vi "Apply New Configuration File.vi"(8 "error in (no error)":errorcluster, 9 "MD5 Hash In":string, 10 "File Path In":path, 11 "CD Ref In":T1=18446744073709551615 format="%.0x") -> (0 "error out":errorcluster, 1 "MD5 Hash Out":string, 2 "File Path Out":path, 3 "Last File content":string)   [LabVIEW 2021, in "Modbus System Explorer.lvlib"]
uses:
  Modbus System Explorer.lvlib
  <vilib>/NI VeriStand/Custom Device API/Custom Device Item Ref.ctl
  Shared/3_But_Dlg_Symbol.ctl
  Shared/Modbus GUID Lookup.vi
  <vilib>/NI VeriStand/Custom Device Tools/Custom Device Utility Library/NI VeriStand - Search for All Items by GUID.vi
  Glyphs/Modbus Dialog Messages.vi
  Glyphs/Modbus Property Names.vi
  <vilib>/NI VeriStand/Custom Device API/Get Item Property (String).vi
  <vilib>/NI VeriStand/Custom Device API/Get Item Property (Path).vi
  <vilib>/NI VeriStand/Custom Device API/Set Item Property (Variant).vi
  <vilib>/NI VeriStand/Custom Device API/Set Item Property (Path).vi
  <vilib>/NI VeriStand/Custom Device API/Set Item Property (String).vi
  Shared/Modbus Shared.lvlib
  <vilib>/NI VeriStand/Custom Device API/Custom Device API.lvlib
  XML Deserializer/XML VIs/API/XML_Deserializer.lvlib
  <vilib>/NI VeriStand/Custom Device Tools/Custom Device Utility Library/Custom Device Utility Library.lvlib
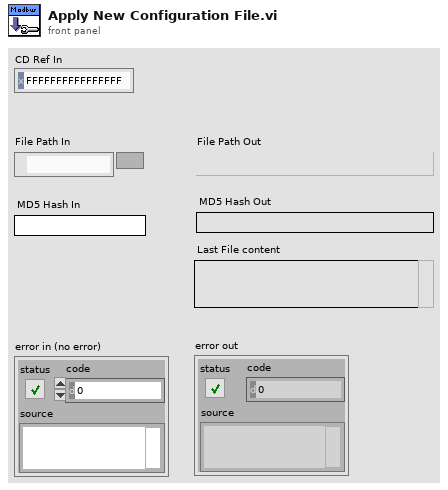
[diagram p1: front panel]
types:
  T1 = typedef "Custom Device API.lvlib/Custom Device Item Ref.ctl" = u64
  T2 = typedef "Modbus Shared.lvlib/3_But_Dlg_Symbol.ctl" = enum16{"Information", "Help", "Warning", "Error"}
  T3 = typedef "Modbus Shared.lvlib/Modbus_General_Settings.ctl" = cluster{"Communication_Type":T4, "Modbus_Type":T5, "Read_Write_Loop_Period":i64, "TCP Settings":cluster{"TCP_Settings_Port":u16, "TCP_Settings_IP_Timeout":u32, "TCP_Settings_IP_Slave_Address":string}, "Serial Settings":cluster{"Serial_Settings_Flow_Control":T6, "Serial_Settings_Baud_Rate":u32, "Serial_Settings_Parity":T7, "Serial_Settings_Resource_Name":string, "Serial_Settings_Serial_Type":T8, "Serial_Settings_Unit_ID":u8}}
  T4 = typedef "Modbus Shared.lvlib/Modbus_Communication_Type.ctl" = i32
  T5 = typedef "Modbus Shared.lvlib/Modbus_Type.ctl" = i32
  T6 = typedef "Modbus Shared.lvlib/Modbus_Serial_Settings_Flow_Control.ctl" = i32
  T7 = typedef "Modbus Shared.lvlib/Modbus_Serial_Settings_Parity.ctl" = i32
  T8 = typedef "Modbus Shared.lvlib/Modbus_Serial_Settings_Serial_Type.ctl" = i32
  T9 = typedef "Modbus Shared.lvlib/Modbus_Items.ctl" = cluster{"Modbus Type":T10, "Base Name":string, "Starting Address":u16, "Quantity":u16}
  T10 = typedef "Modbus Shared.lvlib/Modbus_Item_Type.ctl" = enum16{"Read Coils", "Read Discrete Inputs", "Read Holding Registers", "Read Input Registers", "Write Multiple Coils", "Write Multiple Holding Registers", "Write Single Coil", "Write Single Holding Register", "Write Multiple Discrete Inputs", "Write Multiple Input Registers"}
  T11 = typedef "Modbus Shared.lvlib/Channels Ref.ctl" = cluster{"Array of Refs":T1[]}
  T12 = typedef "Modbus Shared.lvlib/FIFO Indexes.ctl" = cluster{"FIFO Indexes":i32[], "FIFO Buffer":T13}
  T13 = typedef "Custom Device API.lvlib/Custom Device Channel Type.ctl" = enum16{"Input", "Output"}
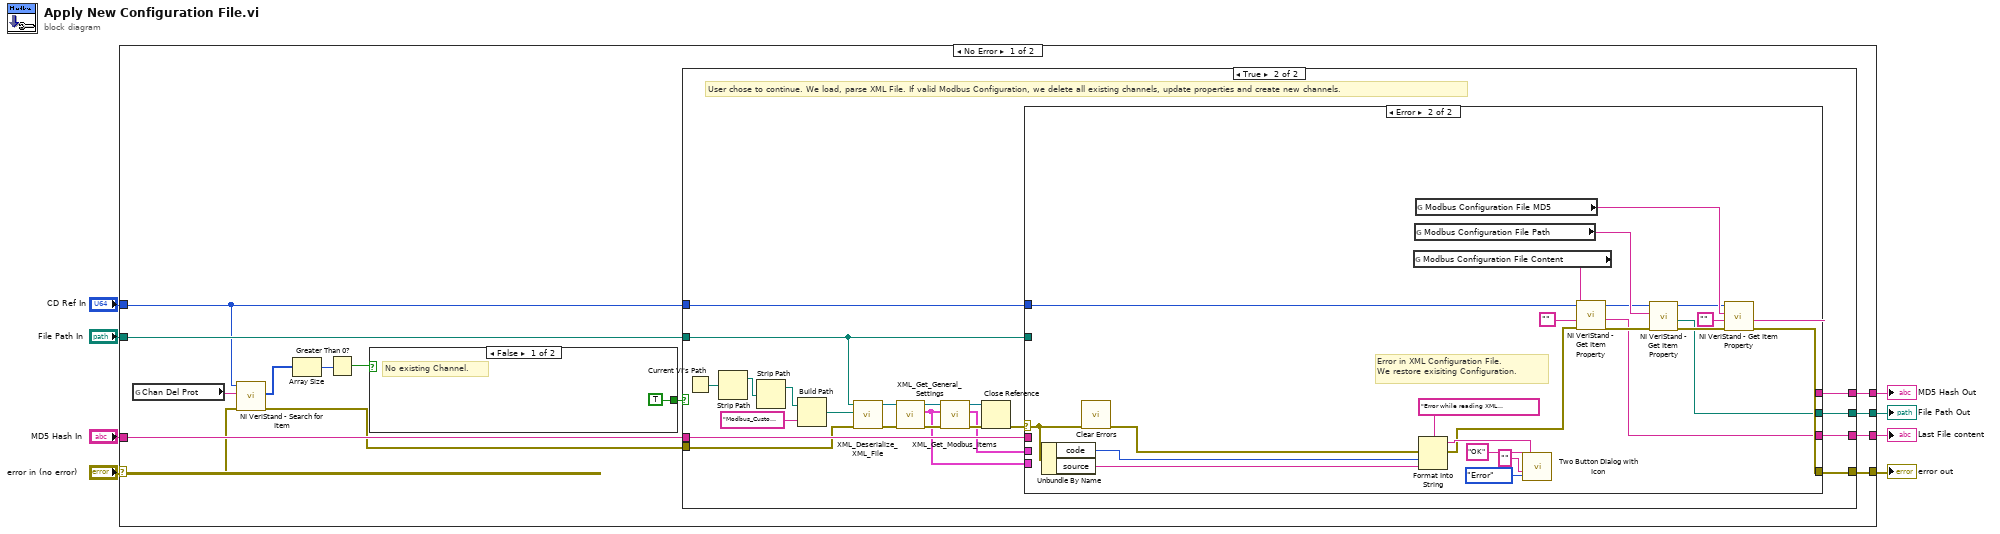
[diagram p0: block diagram]
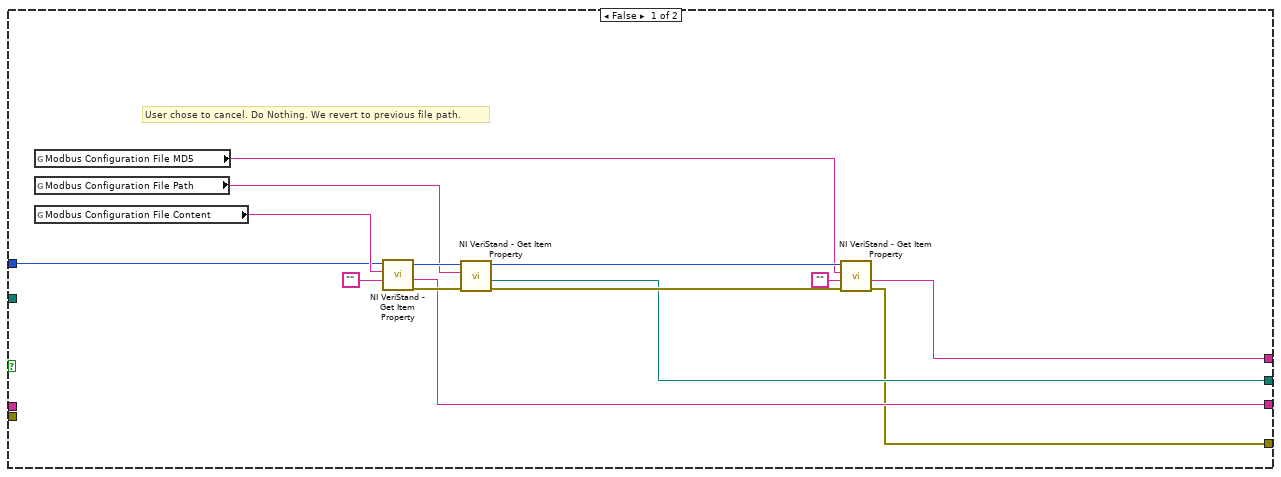
[diagram p2: hidden frame]
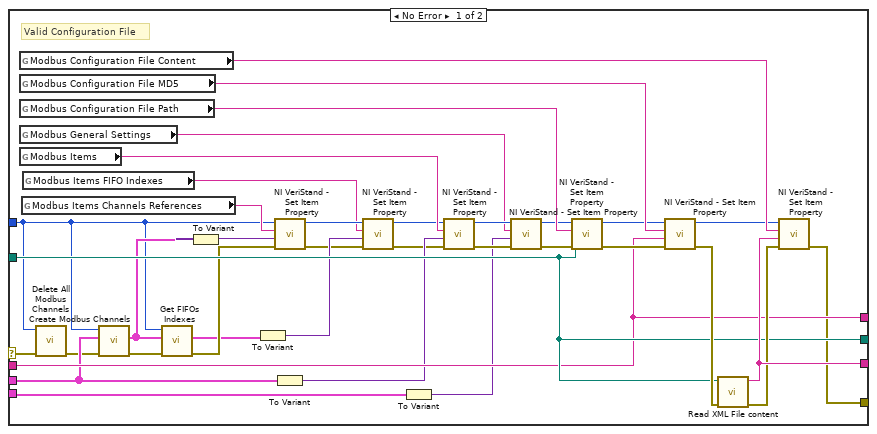
[diagram p3: hidden frame]
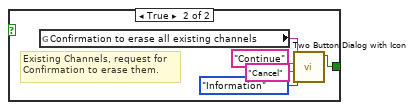
[diagram p4: hidden frame]
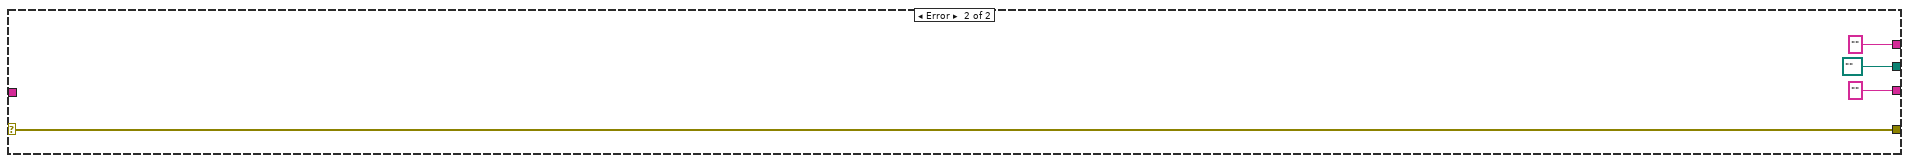
[diagram p5: hidden frame]
diagram:
  n1 = case shown="No Error" "error in (no error)" {
    selector: "error in (no error)" -> [w13 w129]
    tunnel: [w17 w129] -> w7
    tunnel: "CD Ref In" -> [w14 _]
    tunnel: "File Path In" -> [w21 _]
    tunnel: [w20 "" ("MD5 Hash In")] -> w4
    tunnel: [w19 path "" ("File Path In")] -> w3
    tunnel: [w18 "" ("XML File content")] -> w2
    tunnel: "MD5 Hash In" -> [w16 _]
    frame No Error {
      n2 = global read "Modbus GUID Lookup.vi" "Chan Del Prot"() -> (w15:string)
      n3 = call-poly <vilib>:"NI VeriStand - Search for Item.vi"("error in"=w13, "Item GUID"=w15, "Section Ref in"=w14) -> ("error out"=w9:errorcluster, "Item Refs"=w12:T1[])  [unwired: 5 in, 2 out]
      n4 = Array Size(array=w12) -> (size(s)=w11:i32)
      n5 = Greater Than 0?(x=w11) -> (x > 0?=w10:bool)
      n6 = case shown="False" w10 {
        tunnel: [TRUE ("T button?") w124] -> w22
        frame False {
          # "No existing Channel."
        }
        frame True {
          # "Existing Channels, request for\nConfirmation to erase them."
          n7 = global read "Modbus Dialog Messages.vi" "Confirmation to erase all existing channels"() -> (w123:string)
          n8 = call "Two Button Dialog with Icon.vi"("Symbol"=3_But_Dlg_Symbol."Information", "F button name (\"Cancel\")"="Cancel" ("F button name (\"Cancel\")"), "T button name (\"OK\")"="Continue" ("T button name (\"OK\")"), "Message"=w123) -> ("T Button?"=w124:bool)  [unwired: 7 in]
        }
      }
      n9 = case shown="True" w22 {
        tunnel: w14 -> [w28 w55]
        tunnel: w21 -> [_ w45]
        tunnel: [w27 w53] -> w20
        tunnel: [w26 w54] -> w19
        tunnel: [w25 w58] -> w18
        tunnel: [w24 w56] -> w17
        tunnel: w16 -> [_ w57]
        tunnel: w9 -> [_ w37]
        frame False {
          # "User chose to cancel. Do Nothing. We revert to previous file path."
          n10 = global read "Modbus Property Names.vi" "Modbus Configuration File MD5"() -> (w31:string)
          n11 = global read "Modbus Property Names.vi" "Modbus Configuration File Path"() -> (w32:string)
          n12 = global read "Modbus Property Names.vi" "Modbus Configuration File Content"() -> (w30:string)
          n13 = call-poly <vilib>:"NI VeriStand - Get Item Property.vi"("Default Value"="", "Property Name"=w30, "Item Ref in"=w28) -> ("error out"=w36:errorcluster, "Value"=w25:string, "Item Ref out"=w33:T1)  [unwired: 5 in, 1 out]
          n14 = call-poly <vilib>:"NI VeriStand - Get Item Property.vi"("error in (no error)"=w36, "Property Name"=w32, "Item Ref in"=w33) -> ("error out"=w35:errorcluster, "Value"=w26:path, "Item Ref out"=w34:T1)  [unwired: 5 in, 1 out]
          n15 = call-poly <vilib>:"NI VeriStand - Get Item Property.vi"("error in (no error)"=w35, "Default Value"="", "Property Name"=w31, "Item Ref in"=w34) -> ("error out"=w24:errorcluster, "Value"=w27:string)  [unwired: 4 in, 2 out]
        }
        frame True {
          # "User chose to continue. We load, parse XML File. If valid Modbus Configuration, we delete all existing channels, update properties and create new channels."
          n16 = Current VI's Path() -> (path=w41:path)
          n17 = Strip Path(path=w41) -> (stripped path=w40:path)  [unwired: 1 out]
          n18 = Strip Path(path=w40) -> (stripped path=w39:path)  [unwired: 1 out]
          n19 = Build Path(base path=w39, name or relative path="Modbus_Custom_Device.xsd") -> (appended path=w43:path)
          n20 = call "XML_Deserialize_XML_File.vi"("error in (no error)"=w37, "XSD Path"=w43, "XML Path"=w45) -> ("error out"=w51:errorcluster, "reference out"=w52:refnum<k24>)  [unwired: 7 in]
          n21 = call "XML_Get_General_Settings.vi"("error in (no error)"=w51, ".NET Refnum in"=w52) -> ("error out"=w49:errorcluster, "General Settings"=w42:T3, ".NET Refnum out"=w50:refnum<k24>)  [unwired: 7 in]
          n22 = call "XML_Get_Modbus_Items.vi"("error in (no error)"=w49, "General Settings"=w42, "reference out"=w50) -> ("error out"=w48:errorcluster, "Array"=w44:T9[], "reference out"=w47:refnum<k24>)  [unwired: 6 in]
          n23 = Close Reference(reference=w47, error in (no error)=w48) -> (error out=w46:errorcluster)
          n24 = case shown="Error" w46 {
            selector: w46 -> [w85 w104]
            tunnel: [w94 w108] -> w58
            tunnel: w57 -> [w80 _]
            tunnel: w45 -> [w86 _]
            tunnel: [w70 w109] -> w56
            tunnel: w55 -> [w66 w110]
            tunnel: [w86 w106] -> w54
            tunnel: [w80 w107] -> w53
            tunnel: w44 -> [w76 _]
            tunnel: w42 -> [w78 _]
            frame No Error {
              # "Valid Configuration File"
              n25 = global read "Modbus Property Names.vi" "Modbus Configuration File Content"() -> (w95:string)
              n26 = global read "Modbus Property Names.vi" "Modbus Configuration File MD5"() -> (w93:string)
              n27 = global read "Modbus Property Names.vi" "Modbus Configuration File Path"() -> (w87:string)
              n28 = global read "Modbus Property Names.vi" "Modbus General Settings"() -> (w74:string)
              n29 = global read "Modbus Property Names.vi" "Modbus Items"() -> (w73:string)
              n30 = global read "Modbus Property Names.vi" "Modbus Items Channels References"() -> (w72:string)
              n31 = global read "Modbus Property Names.vi" "Modbus Items FIFO Indexes"() -> (w60:string)
              n32 = call "Delete All Modbus Channels.vi"("error in (no error)"=w85, "CD Ref In"=w66) -> ("error out"=w75:errorcluster)  [unwired: 9 in]
              n33 = call "Create Modbus Channels.vi"("error in (no error)"=w75, "Array"=w76, "CD Ref In"=w66) -> ("error out"=w68:errorcluster, "Channels Refs"=w69:T11[])  [unwired: 7 in]
              n34 = call "Get FIFOs Indexes.vi"("error in (no error)"=w68, "Channels Refs"=w69, "Device Ref in"=w66) -> ("error out"=w67:errorcluster, "Array"=w59:T12[])  [unwired: 7 in]
              n35 = To Variant(anything=w69) -> (Variant=w71:variant)
              n36 = To Variant(anything=w59) -> (Variant=w65:variant)
              n37 = call-poly <vilib>:"NI VeriStand - Set Item Property.vi"("error in (no error)"=w67, "Value"=w71, "Property Name"=w72, "Item Ref in"=w66) -> ("error out"=w62:errorcluster, "Item Ref out"=w64:T1)  [unwired: 5 in, 1 out]
              n38 = To Variant(anything=w76) -> (Variant=w79:variant)
              n39 = call-poly <vilib>:"NI VeriStand - Set Item Property.vi"("error in (no error)"=w62, "Value"=w65, "Property Name"=w60, "Item Ref in"=w64) -> ("error out"=w61:errorcluster, "Item Ref out"=w63:T1)  [unwired: 5 in, 1 out]
              n40 = To Variant(anything=w78) -> (Variant=w77:variant)
              n41 = call-poly <vilib>:"NI VeriStand - Set Item Property.vi"("error in (no error)"=w61, "Value"=w79, "Property Name"=w73, "Item Ref in"=w63) -> ("error out"=w84:errorcluster, "Item Ref out"=w81:T1)  [unwired: 5 in, 1 out]
              n42 = call-poly <vilib>:"NI VeriStand - Set Item Property.vi"("error in (no error)"=w84, "Value"=w77, "Property Name"=w74, "Item Ref in"=w81) -> ("error out"=w83:errorcluster, "Item Ref out"=w82:T1)  [unwired: 5 in, 1 out]
              n43 = call-poly <vilib>:"NI VeriStand - Set Item Property.vi"("error in (no error)"=w83, "Value"=w86, "Property Name"=w87, "Item Ref in"=w82) -> ("error out"=w88:errorcluster, "Item Ref out"=w89:T1)  [unwired: 5 in, 1 out]
              n44 = call-poly <vilib>:"NI VeriStand - Set Item Property.vi"("error in (no error)"=w88, "Value"=w80, "Property Name"=w93, "Item Ref in"=w89) -> ("error out"=w91:errorcluster, "Item Ref out"=w92:T1)  [unwired: 5 in, 1 out]
              n45 = call "Read XML File content.vi"("error in (no error)"=w91, "Path"=w86) -> ("error out"=w90:errorcluster, "XML File content"=w94:string)  [unwired: 8 in]
              n46 = call-poly <vilib>:"NI VeriStand - Set Item Property.vi"("error in (no error)"=w90, "Value"=w94, "Property Name"=w95, "Item Ref in"=w92) -> ("error out"=w70:errorcluster)  [unwired: 5 in, 2 out]
            }
            frame Error {
              # "Error in XML Configuration File.\nWe restore exisiting Configuration."
              n47 = Unbundle By Name(w104) -> ("code"=w103:i32, "source"=w102:string)
              n48 = call <vilib>:"Clear Errors.vi"("error in (no error)"=w104) -> ("error out"=w105:errorcluster)  [unwired: 5 in, 1 out]
              n49 = global read "Modbus Property Names.vi" "Modbus Configuration File Content"() -> (w117:string)
              n50 = global read "Modbus Property Names.vi" "Modbus Configuration File Path"() -> (w115:string)
              n51 = global read "Modbus Property Names.vi" "Modbus Configuration File MD5"() -> (w116:string)
              n52 = Format Into String(format string="Error while reading XML Configuration File: \nError: %d\nMessage: %s", error in=w105, w103, w102) -> (resulting string=w100:string, error out=w96:errorcluster)  [unwired: 1 in]
              n53 = call "Two Button Dialog with Icon.vi"("Symbol"=3_But_Dlg_Symbol."Error", "F button name (\"Cancel\")"="" ("F button name (\"Cancel\")"), "T button name (\"OK\")"="OK" ("T button name (\"OK\")"), "Message"=w100) -> ()  [unwired: 7 in, 1 out]
              n54 = call-poly <vilib>:"NI VeriStand - Get Item Property.vi"("error in (no error)"=w96, "Default Value"="", "Property Name"=w117, "Item Ref in"=w110) -> ("error out"=w111:errorcluster, "Value"=w108:string, "Item Ref out"=w114:T1)  [unwired: 4 in, 1 out]
              n55 = call-poly <vilib>:"NI VeriStand - Get Item Property.vi"("error in (no error)"=w111, "Property Name"=w115, "Item Ref in"=w114) -> ("error out"=w112:errorcluster, "Value"=w106:path, "Item Ref out"=w113:T1)  [unwired: 5 in, 1 out]
              n56 = call-poly <vilib>:"NI VeriStand - Get Item Property.vi"("error in (no error)"=w112, "Default Value"="", "Property Name"=w116, "Item Ref in"=w113) -> ("error out"=w109:errorcluster, "Value"=w107:string)  [unwired: 4 in, 2 out]
            }
          }
        }
      }
    }
    frame Error {
    }
  }
  "File Path Out" <- w3
  "MD5 Hash Out" <- w4
  "Last File content" <- w2
  "error out" <- w7
